vi "Write Output_Enable.vi"(8 "error in":errorcluster, 10 "Output_Enable":bool, 11 "6032A in":refnum<class "6032A.lvclass">) -> (0 "error out":errorcluster, 3 "6032A out":refnum<class "6032A.lvclass">)   [LabVIEW 2019, in "6032A.lvlib" / "6032A.lvclass"]
uses:
  Library/6032A.lvclass
  Library/6032A.lvclass/6032A.ctl
  builds/Instruments/PowerSupply.lvlibp/Library/PowerSupply.lvclass
  <instrlib>/Agilent 6XXX Series/Agilent 6XXX Series.lvlib
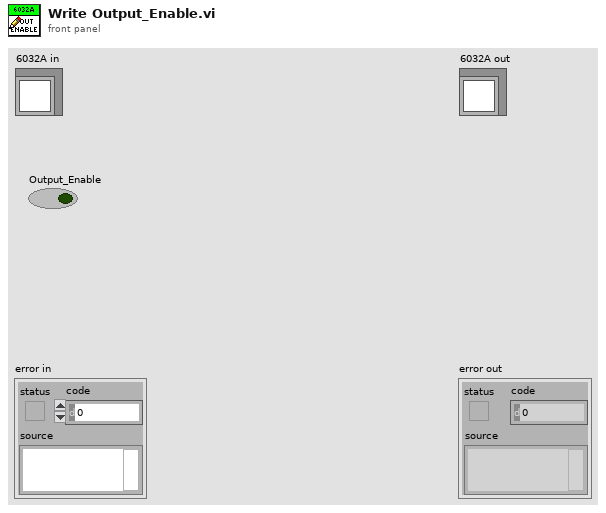
[diagram p1: front panel]
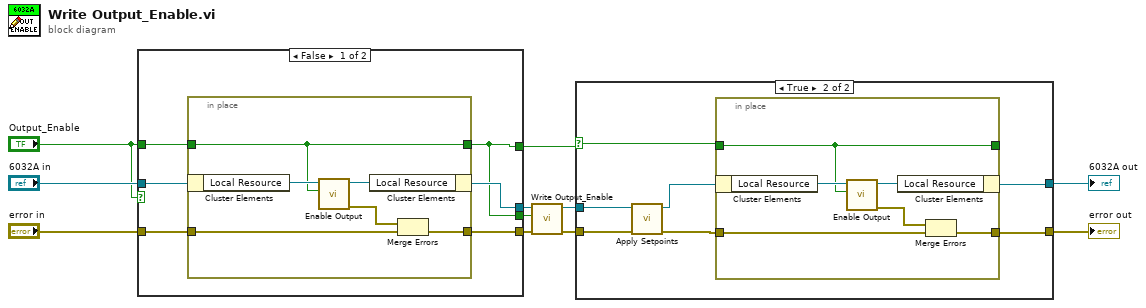
[diagram p0: block diagram]
diagram:
  n1 = case shown="False" "Output_Enable" {
    tunnel: "6032A in" -> [w17 w26]
    tunnel: [w16 w26] -> w10
    tunnel: [w15 w25] -> w9
    tunnel: "error in" -> [w14 w25]
    tunnel: "Output_Enable" -> [w13 w24]
    tunnel: [w12 w24] -> w7
    tunnel: [w12 w24] -> w5
    frame False {
      n2 = in-place {
        in-place-border: [w19] -> w15
        in-place-border: w14 -> [w18]
        in-place-border: w13 -> [w20]
        in-place-border: [w20] -> w12
        n3 = in-place-cluster #1(w17) -> ("Local Resource"=w23:refnum<visa-resource-name>)
        n4 = call <instrlib>:"Enable Output.vi"("output (T:on)"=w20, "VISA resource name"=w23) -> ("error out"=w21:errorcluster, "VISA resource name out"=w22:refnum<visa-resource-name>)  [unwired: 8 in]
        n5 = in-place-cluster #1("Local Resource"=w22) -> (w16:refnum<class "6032A.lvclass">)
        n6 = Merge Errors(w21, w18) -> (w19:errorcluster)
      }
    }
    frame True {
    }
  }
  n7 = call-parent "Write Output_Enable.vi"("error in"=w9, "Output_Enable"=w7, "PowerSupply in"=w10) -> ("error out"=w3:errorcluster, "PowerSupply out"=w4:refnum<class "6032A.lvclass">)  [unwired: 7 in]
  n8 = case shown="True" w5 {
    selector: w5 -> [_ w33]
    tunnel: w4 -> [w28 w34]
    tunnel: w3 -> [w27 w35]
    tunnel: [w27 w29] -> w2
    tunnel: [w28 w30] -> w1
    frame False {
    }
    frame True {
      n9 = call "Apply Setpoints.vi"("error in"=w35, "6032A in"=w34) -> ("error out"=w31:errorcluster, "6032A out"=w32:refnum<class "6032A.lvclass">)  [unwired: 8 in]
      n10 = in-place {
        in-place-border: [w37] -> w29
        in-place-border: w31 -> [w36]
        in-place-border: w33 -> [w38]
        in-place-border: [w38] -> _
        n11 = in-place-cluster #2(w32) -> ("Local Resource"=w41:refnum<visa-resource-name>)
        n12 = call <instrlib>:"Enable Output.vi"("output (T:on)"=w38, "VISA resource name"=w41) -> ("error out"=w39:errorcluster, "VISA resource name out"=w40:refnum<visa-resource-name>)  [unwired: 8 in]
        n13 = in-place-cluster #2("Local Resource"=w40) -> (w30:refnum<class "6032A.lvclass">)
        n14 = Merge Errors(w39, w36) -> (w37:errorcluster)
      }
    }
  }
  "error out" <- w2
  "6032A out" <- w1
